vi "Configure Relative Reading.vi"(0 "VISA resource name":refnum<visa-resource-name>, 1 "Enable Relative Reading (F: Disable)":bool, 5 "Relative Data Feed (0: Input Signal)":u16(ring) items=["Input Signal", "Math Result"], 7 "Offset Value (0)":dbl, 11 "error in (no error)":errorcluster) -> (4 "VISA resource name out":refnum<visa-resource-name>, 15 "error out":errorcluster)   [LabVIEW 2020, in "Keithley 648X Series.lvlib"]
doc: "Configures the relative reading calculation.\n\n<b>Note:</b>\nThis VI only allows you to set a constant as the offset value for the relative function. To acquire a value based on the instrument setup use the <b>Acquire Relative Offset</b> action VI."
uses:
  <instrlib>/Keithley 648X Series/Keithley 648X Series.lvlib
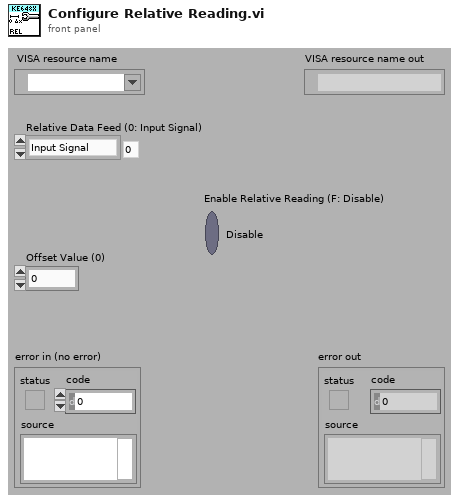
[diagram p1: front panel]
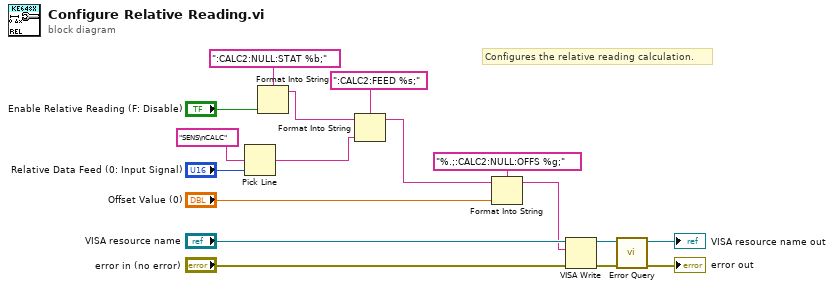
[diagram p0: block diagram]
diagram:
  # "Configures the relative reading calculation."
  n1 = Pick Line(multi-line string="SENS\nCALC", line index="Relative Data Feed (0: Input Signal)") -> (output string=w6:string)  [unwired: 1 in]
  n2 = Format Into String(format string=":CALC2:NULL:STAT %b;", "Enable Relative Reading (F: Disable)") -> (resulting string=w5:string)  [unwired: 2 in, 1 out]
  n3 = Format Into String(format string=":CALC2:FEED %s;", initial string=w5, w6) -> (resulting string=w4:string)  [unwired: 1 in, 1 out]
  n4 = Format Into String(format string="%.;:CALC2:NULL:OFFS %g;", initial string=w4, "Offset Value (0)") -> (resulting string=w2:string)  [unwired: 1 in, 1 out]
  n5 = VISA Write(VISA resource name="VISA resource name", write buffer=w2, error in (no error)="error in (no error)") -> (VISA resource name out=w13:refnum<visa-resource-name>, error out=w12:errorcluster)  [unwired: 1 out]
  n6 = call <instrlib>:"Error Query.vi"("error in (no error)"=w12, "VISA resource name"=w13) -> ("error out"=→"error out":errorcluster, "VISA resource name out"=→"VISA resource name out":refnum<visa-resource-name>)  [unwired: 6 in, 2 out]
